vi "Write Spectral Data (SubVI).vi"(0 "Measurement Cluster IN":T1, 3 "ON/OFF IN":bool, 4 "Write Spectral Data":bool, 5 "Measurement Mode IN":enum32{"Emission", "Absorption"}(radio), 7 "File Path IN":path, 9 "Run Info":string, 11 "NSave":i32) -> (14 "Measurement Cluster OUT":T1, 18 "Reset Write Spectral Data":bool, 19 "Write Progress":u8)   [LabVIEW 2018]
uses:
  Measurement Cluster.ctl
  <vilib>/Utility/file.llb/Write Delimited Spreadsheet (string).vi
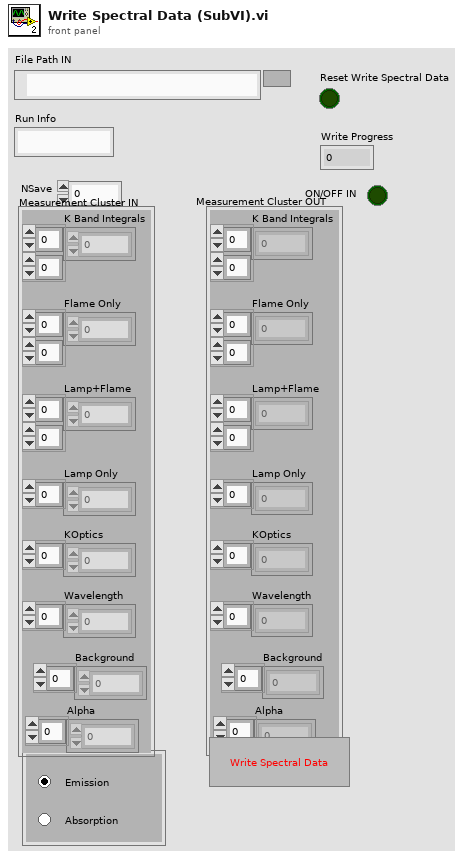
[diagram p1: front panel]
types:
  T1 = typedef "Measurement Cluster.ctl" = cluster{"K Band Integrals":dbl[][], "Flame Only":dbl[][], "Lamp+Flame":dbl[][], "Lamp Only":dbl[], "KOptics":dbl[], "Wavelength":dbl[], "Background":dbl[], "Alpha":dbl[]}
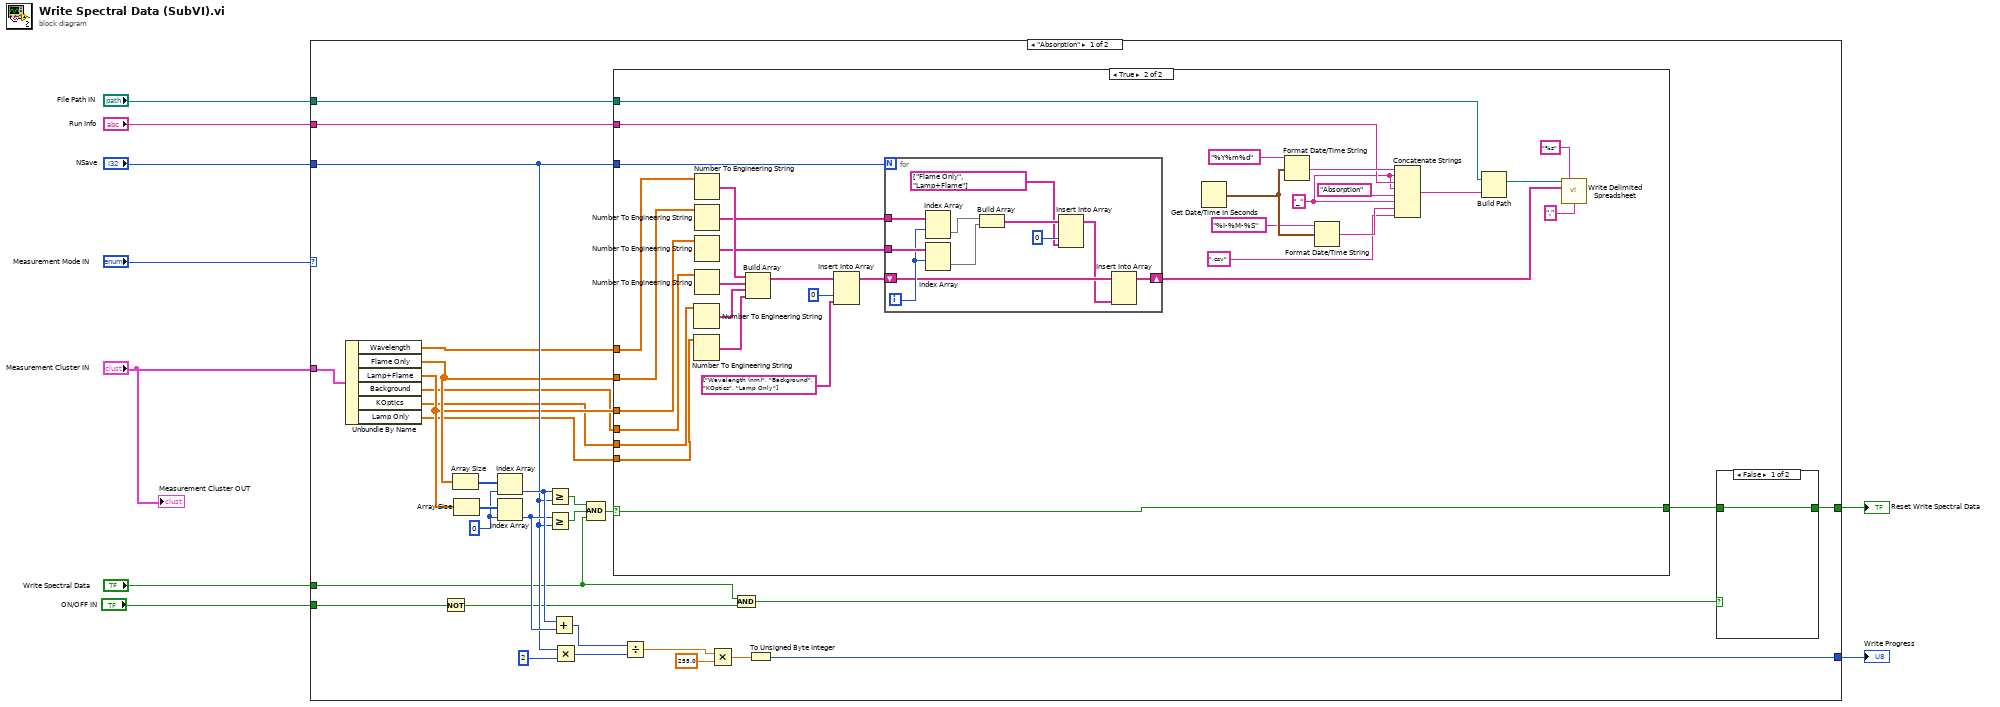
[diagram p0: block diagram]
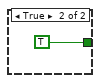
[diagram p2: hidden frame]
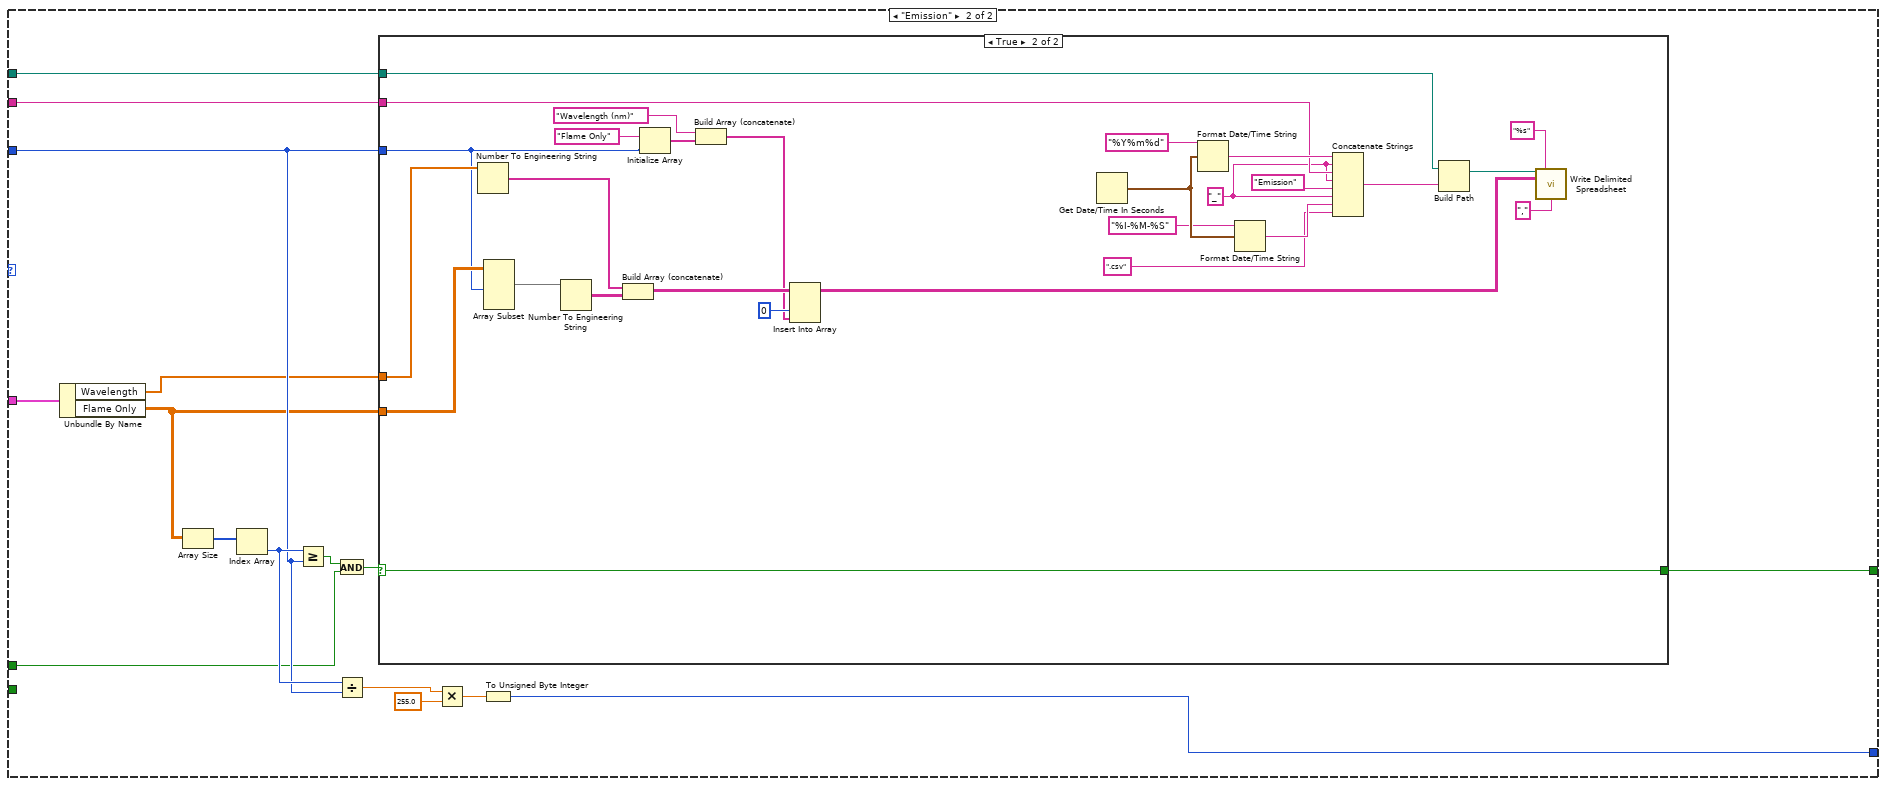
[diagram p4: hidden frame]
diagram:
  n1 = case shown="\"Absorption\"" "Measurement Mode IN" {
    tunnel: "NSave" -> [w30 w98]
    tunnel: "File Path IN" -> [w34 w102]
    tunnel: "Run Info" -> [w33 w101]
    tunnel: [w13 w100] -> w8
    tunnel: [w23 w94] -> w7
    tunnel: "Measurement Cluster IN" -> [w22 w93]
    tunnel: "Write Spectral Data" -> [w16 w88]
    tunnel: "ON/OFF IN" -> [w17 _]
    frame "Absorption" {
      w38 = 0 ("index")
      n2 = Unbundle By Name(w22) -> ("Wavelength"=w21:dbl[], "Flame Only"=w20:dbl[][], "Lamp+Flame"=w19:dbl[][], "Background"=w18:dbl[], "KOptics"=w11:dbl[], "Lamp Only"=w10:dbl[])
      n3 = Not(x=w17) -> (.not. x?=w15:bool)
      n4 = Array Size(array=w20) -> (size(s)=w40:i32[])
      n5 = Array Size(array=w19) -> (size(s)=w39:i32[])
      n6 = Index Array(array=w40, index=w38) -> (element=w32:i32)
      n7 = Index Array(array=w39, index=w38) -> (element=w31:i32)
      n8 = Greater Or Equal?(x=w32, y=w30) -> (x >= y?=w37:bool)
      n9 = Greater Or Equal?(x=w31, y=w30) -> (x >= y?=w36:bool)
      n10 = Add(x=w32, y=w31) -> (x+y=w28:i32)
      n11 = Multiply(x=w30, y=2) -> (x*y=w27:i32)
      n12 = Compound Arithmetic op=AND(w37, w36, w16) -> (w35:bool)
      n13 = case shown="True" w35 {
        selector: w35 -> [w43 w49]
        tunnel: w30 -> [_ w69]
        tunnel: w21 -> [_ w67]
        tunnel: w20 -> [_ w66]
        tunnel: w19 -> [_ w65]
        tunnel: w18 -> [_ w46]
        tunnel: w34 -> [_ w54]
        tunnel: w33 -> [_ w51]
        tunnel: [w43 w49] -> w12
        tunnel: w11 -> [_ w45]
        tunnel: w10 -> [_ w44]
        frame False {
        }
        frame True {
          w50 = "_"
          n14 = Number To Engineering String(4:w45) -> (0:w48:string[])  [unwired: 3 in]
          n15 = Number To Engineering String(4:w44) -> (0:w47:string[])  [unwired: 3 in]
          n16 = Number To Engineering String(4:w67) -> (0:w76:string[])  [unwired: 3 in]
          n17 = Number To Engineering String(4:w66) -> (0:w74:string[][])  [unwired: 3 in]
          n18 = Number To Engineering String(4:w65) -> (0:w73:string[][])  [unwired: 3 in]
          n19 = Number To Engineering String(4:w46) -> (0:w75:string[])  [unwired: 3 in]
          n20 = Build Array(w76, w75, w48, w47) -> (w72:string[][])
          n21 = Insert Into Array(array=w72, index (col)=0 ("index (row)"), new element=string[] ["Wavelength (nm)", "Background", "KOptics", "Lamp Only"]) -> (w68:string[][])  [unwired: 1 in]
          n22 = for {
            N: w69 -> [_]
            tunnel: w74 -> [w86]
            tunnel: w73 -> [w85]
            shift-right: [w77] -> w55
            shift-left: w68 -> [w79]
            i -> [w84]
            n23 = Index Array(array=w86, index (row)=w84) -> (element=w83:string[])  [unwired: 1 in]
            n24 = Index Array(array=w85, index (row)=w84) -> (element=w82:string[])  [unwired: 1 in]
            n25 = Build Array(w83, w82) -> (w81:string[][])
            n26 = Insert Into Array(array=w81, index (col)=0 ("index (row)"), new element=string[] ["Flame Only", "Lamp+Flame"]) -> (w78:string[][])  [unwired: 1 in]
            n27 = Insert Into Array(array=w79, new element=w78) -> (w77:string[][])  [unwired: 2 in]
          }
          n28 = Get Date/Time In Seconds() -> (seconds since 1Jan1904=w64:timestamp)
          n29 = Format Date/Time String(time format string (%c)="%Y%m%d", seconds (now)=w64) -> (date/time string=w53:string)  [unwired: 1 in]
          n30 = Format Date/Time String(time format string (%c)="%I-%M-%S", seconds (now)=w64) -> (date/time string=w60:string)  [unwired: 1 in]
          n31 = Concatenate Strings(w53, w50, w51, w50, "Absorption" ("time format string (%c)"), w50, w60, ".csv") -> (w61:string)
          n32 = Build Path(base path=w54, name or relative path=w61) -> (appended path=w56:path)
          n33 = call-poly <vilib>:"Write Delimited Spreadsheet.vi"("file path (dialog if empty)"=w56, "format (%s)"="%s" ("format (%.3f)"), "2D data"=w55, "delimiter (\\t)"="," ("delimiter (\\t)")) -> ()  [unwired: 10 in, 2 out]
        }
      }
      n34 = Divide(x=w28, y=w27) -> (x/y=w24:dbl)
      n35 = Multiply(x=w24, y=255.0) -> (x*y=w26:dbl)
      n36 = And(x=w16, y=w15) -> (x .and. y?=w14:bool)
      n37 = To Unsigned Byte Integer(number=w26) -> (unsigned 8bit integer=w23:u8)
      n38 = case shown="False" w14 {
        tunnel: [w41 TRUE] -> w13
        tunnel: w12 -> [w41 _]
        frame False {
        }
        frame True {
        }
      }
    }
    frame "Emission" {
      n39 = Unbundle By Name(w93) -> ("Wavelength"=w92:dbl[], "Flame Only"=w91:dbl[][])
      n40 = Array Size(array=w91) -> (size(s)=w103:i32[])
      n41 = Index Array(array=w103) -> (element=w99:i32)  [unwired: 1 in]
      n42 = Greater Or Equal?(x=w99, y=w98) -> (x >= y?=w89:bool)
      n43 = And(x=w89, y=w88) -> (x .and. y?=w90:bool)
      n44 = Divide(x=w99, y=w98) -> (x/y=w96:dbl)
      n45 = case shown="True" w90 {
        selector: w90 -> [w104 w105]
        tunnel: w98 -> [_ w107]
        tunnel: w92 -> [_ w128]
        tunnel: w91 -> [_ w108]
        tunnel: w102 -> [_ w118]
        tunnel: w101 -> [_ w115]
        tunnel: [w104 w105] -> w100
        frame False {
        }
        frame True {
          w114 = "_"
          n46 = Number To Engineering String(4:w128) -> (0:w132:string[])  [unwired: 3 in]
          n47 = Array Subset(array=w108, length (row)=w107) -> (w106:dbl[][])  [unwired: 3 in]
          n48 = Number To Engineering String(4:w106) -> (0:w131:string[][])  [unwired: 3 in]
          n49 = Build Array (concatenate)(w132, w131) -> (w130:string[][])
          n50 = Initialize Array("Flame Only", w107) -> (w111:string[])
          n51 = Build Array (concatenate)("Wavelength (nm)", w111) -> (w109:string[])
          n52 = Insert Into Array(array=w130, index (col)=0 ("index (row)"), new element=w109) -> (w110:string[][])  [unwired: 1 in]
          n53 = Get Date/Time In Seconds() -> (seconds since 1Jan1904=w127:timestamp)
          n54 = Format Date/Time String(time format string (%c)="%Y%m%d", seconds (now)=w127) -> (date/time string=w117:string)  [unwired: 1 in]
          n55 = Format Date/Time String(time format string (%c)="%I-%M-%S", seconds (now)=w127) -> (date/time string=w123:string)  [unwired: 1 in]
          n56 = Concatenate Strings(w117, w114, w115, w114, "Emission" ("time format string (%c)"), w114, w123, ".csv") -> (w124:string)
          n57 = Build Path(base path=w118, name or relative path=w124) -> (appended path=w119:path)
          n58 = call-poly <vilib>:"Write Delimited Spreadsheet.vi"("file path (dialog if empty)"=w119, "format (%s)"="%s" ("format (%.3f)"), "2D data"=w110, "delimiter (\\t)"="," ("delimiter (\\t)")) -> ()  [unwired: 10 in, 2 out]
        }
      }
      n59 = Multiply(x=w96, y=255.0) -> (x*y=w95:dbl)
      n60 = To Unsigned Byte Integer(number=w95) -> (unsigned 8bit integer=w94:u8)
    }
  }
  "Reset Write Spectral Data" <- w8
  "Write Progress" <- w7
  "Measurement Cluster OUT" <- "Measurement Cluster IN"
